vi "JSONtoControlValue.vi"(7 "control (for last item)":refnum<vi>, 8 "error in":errorcluster, 9 "Value":T2, 10 "Value in":variant, 11 "control path":T1(array[cluster])) -> (0 "error out":errorcluster, 2 "Value out":variant)   [LabVIEW 2019, in "SetGetControlValue.lvlib"]
uses:
  SetGetControlValue.lvlib
  Variant/VariantArrayAccessMulti.vi
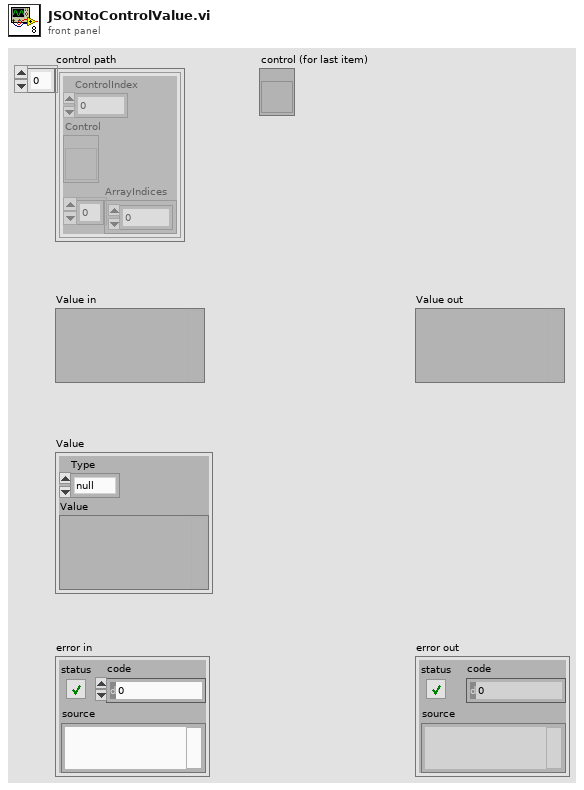
[diagram p1: front panel]
types:
  T1 = cluster{"ControlIndex":i32, "Control":refnum<vi>, "ArrayIndices":i32[]}[]
  T2 = cluster{"Type":enum16{"null", "number", "boolean", "string", "array", "object", ""}, "Value":variant}
  T3 = cluster{"ControlIndex":i32, "Control":refnum<vi>, "ArrayIndices":i32[]}
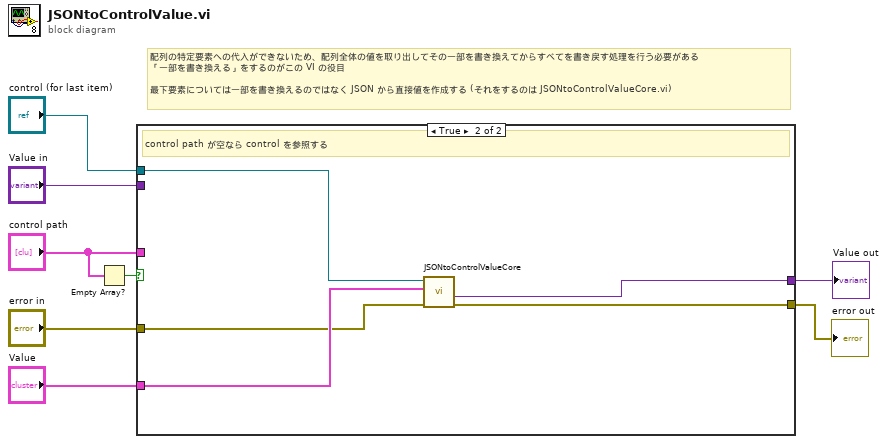
[diagram p0: block diagram]
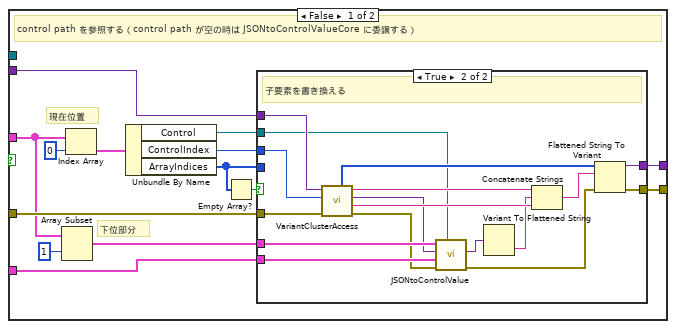
[diagram p2: hidden frame]
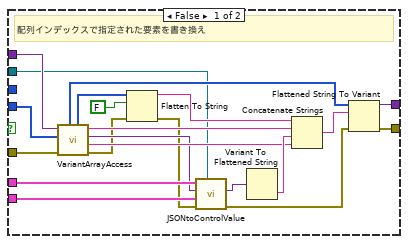
[diagram p3: hidden frame]
diagram:
  # "配列の特定要素への代入ができないため、配列全体の値を取り出してその一部を書き換えてからすべてを書き戻す処理を行う必要がある\n「一部を書き換える」をするのがこの VI の役目\n\n最下要素については一部を書き換えるのではなく JSON から直接値を作成する (それをするのは JSONtoControlValueCore.vi)"
  n1 = Empty Array?(array="control path") -> (empty?=w3:bool)
  n2 = case shown="True" w3 {
    tunnel: [w17 w62] -> w8
    tunnel: "error in" -> [w16 w63]
    tunnel: [w15 w61] -> w6
    tunnel: "Value in" -> [w14 _]
    tunnel: "Value" -> [w11 w64]
    tunnel: "control path" -> [w10 _]
    tunnel: "control (for last item)" -> [_ w65]
    frame False {
      # "下位部分"
      # "現在位置"
      # "control path を参照する（control path が空の時は JSONtoControlValueCore に委譲する）"
      n3 = Array Subset(array=w10, index=1) -> (w19:T1)  [unwired: 1 in]
      n4 = Index Array(array=w10, index=0) -> (element=w9:T3)
      n5 = Unbundle By Name(w9) -> ("Control"=w12:refnum<vi>, "ControlIndex"=w18:i32, "ArrayIndices"=w13:i32[])
      n6 = Empty Array?(array=w13) -> (empty?=w20:bool)
      n7 = case shown="True" w20 {
        tunnel: w19 -> [w40 w57]
        tunnel: w18 -> [_ w45]
        tunnel: w11 -> [w42 w60]
        tunnel: [w41 w59] -> w17
        tunnel: w16 -> [w24 w53]
        tunnel: [w43 w58] -> w15
        tunnel: w14 -> [w26 w54]
        tunnel: w13 -> [w25 _]
        tunnel: w12 -> [w23 w44]
        frame False {
          # "配列インデックスで指定された要素を書き換え"
          n8 = call-poly "VariantArrayAccess.vi"("error in (no error)"=w24, "Indices"=w25, "Array"=w26) -> ("error out"=w28:errorcluster, "rest"=w30:string, "value"=w29:variant, "prepend"=w31:string, "array size"=w35:u32[], "type string"=w36:i16[])  [unwired: 3 in]
          n9 = Flatten To String(anything=w35, prepend array or string size? (T)=FALSE, error in (no error)=w28) -> (data string=w33:string, error out=w27:errorcluster)  [unwired: 1 in, 1 out]
          n10 = call "JSONtoControlValue.vi"("control (for last item)"=w23, "error in"=w27, "Value"=w42, "Value in"=w29, "control path"=w40) -> ("error out"=w38:errorcluster, "Value out"=w37:variant)  [unwired: 5 in]
          n11 = Variant To Flattened String(Variant=w37) -> (data string=w32:string)  [unwired: 1 out]
          n12 = Concatenate Strings(w33, w31, w32, w30) -> (w39:string)
          n13 = Flattened String To Variant(4:w38, 6:w39, 7:w36) -> (0:w43:errorcluster, 3:w41:variant)
        }
        frame True {
          # "子要素を書き換える"
          n14 = call "VariantClusterAccess.vi"("error in (no error)"=w53, "index"=w45, "Cluster Variable"=w54) -> ("error out"=w52:errorcluster, "rest"=w49:string, "value"=w46:variant, "prepend"=w50:string, "type string"=w51:i16[])  [unwired: 4 in]
          n15 = call "JSONtoControlValue.vi"("control (for last item)"=w44, "error in"=w52, "Value"=w60, "Value in"=w46, "control path"=w57) -> ("error out"=w56:errorcluster, "Value out"=w55:variant)  [unwired: 5 in]
          n16 = Variant To Flattened String(Variant=w55) -> (data string=w48:string)  [unwired: 1 out]
          n17 = Concatenate Strings(w50, w48, w49) -> (w47:string)
          n18 = Flattened String To Variant(4:w56, 6:w47, 7:w51) -> (0:w58:errorcluster, 3:w59:variant)
        }
      }
    }
    frame True {
      # "control path が空なら control を参照する"
      n19 = call "JSONtoControlValueCore.vi"("error in"=w63, "Value"=w64, "Control in"=w65) -> ("error out"=w61:errorcluster, "Variant"=w62:variant)  [unwired: 7 in]
    }
  }
  "Value out" <- w8
  "error out" <- w6
